vi "Lookup Child by Name.vi"(8 "error in (no error)":errorcluster, 10 "Child Name":string, 11 "VolatusConfigElement in":refnum<class "VolatusConfigElement.lvclass">) -> (0 "error out":errorcluster, 1 "Found":bool, 2 "Child":refnum<class "Config Element.lvclass">, 3 "VolatusConfigElement out":refnum<class "VolatusConfigElement.lvclass">)   [LabVIEW 2020, in "VolatusConfig.lvlib" / "VolatusConfigElement.lvclass"]
uses:
  VolatusConfigElement.lvclass
  lv-cdm/CDM-Config/Config Element/Config Element.lvclass
  VolatusConfigElement.lvclass/VolatusConfigElement.ctl
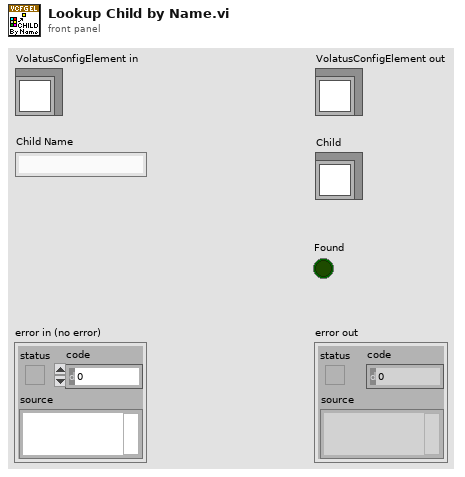
[diagram p1: front panel]
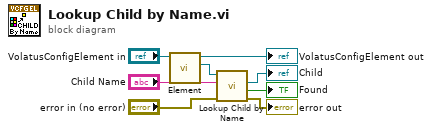
[diagram p0: block diagram]
diagram:
  n1 = call "Element.vi"("VolatusConfigElement in"="VolatusConfigElement in") -> ("Element"=w6:refnum<class "Config Element.lvclass">, "VolatusConfigElement out"=→"VolatusConfigElement out":refnum<class "VolatusConfigElement.lvclass">)  [unwired: 9 in]
  n2 = call "Lookup Child by Name.vi"("error in (no error)"="error in (no error)", "Name"="Child Name", "Config Element in"=w6) -> ("error out"=→"error out":errorcluster, "Found"=→"Found":bool, "Child"=→"Child":refnum<class "Config Element.lvclass">)  [unwired: 5 in, 1 out]
